vi "CameraSetting_DefaultCameraSet.vi"(7 "功能类型":enum16{"读取", "写入"}(ring), 8 "error in (no error)":errorcluster caption="错误输入（无错误）", 9 "CameraBasicInfor":string[](array[string]), 10 "字段名称":string, 11 "configuration file path":path caption="配置文件的路径") -> (0 "error out":errorcluster caption="错误输出")   [LabVIEW 2015]
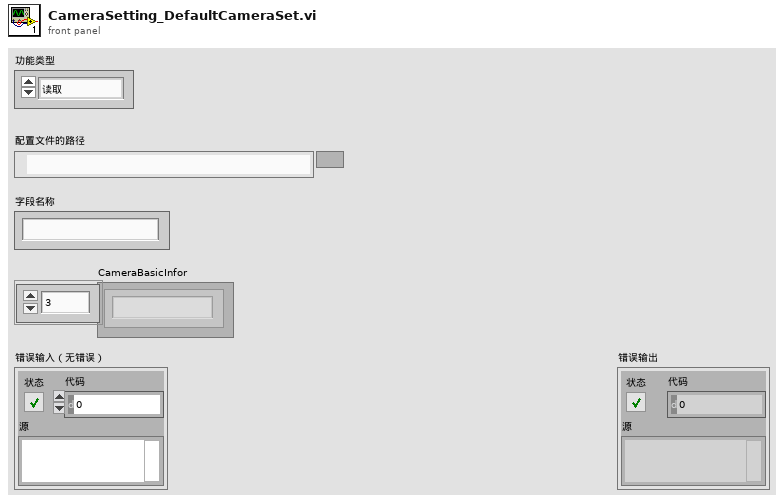
[diagram p1: front panel]
types:
  T1 = enum16{"Boolean", "DBL", "I32", "Path", "String", "U32"}
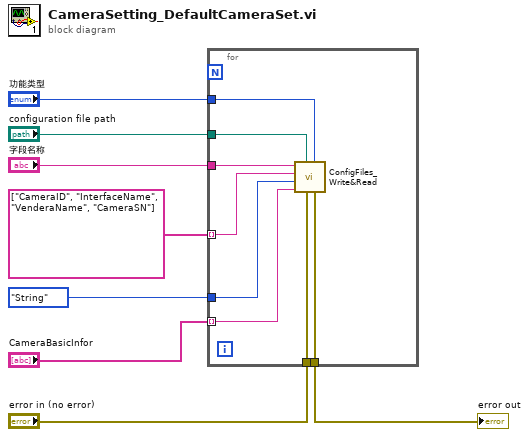
[diagram p0: block diagram]
diagram:
  n1 = for {
    tunnel: "configuration file path" -> [w16]
    tunnel: "功能类型" -> [w15]
    tunnel: "字段名称" -> [w14]
    tunnel: string[] ["CameraID", "InterfaceName", "VenderaName", "CameraSN"] -> [w13] mode=indexing
    tunnel: T1."String" ("键值类型") -> [w12]
    tunnel: "CameraBasicInfor" -> [w11] mode=indexing
    tunnel: "error in (no error)" -> [w10]
    tunnel: [w9] -> w1
    n2 = call "ConfigFiles_Write&Read.vi"("功能类型"=w15, "error in (no error)"=w10, "configuration file path"=w16, "键值_输入"=w11, "键值类型"=w12, "键名称"=w13, "字段名称"=w14) -> ("error out"=w9:errorcluster)  [unwired: 1 in, 3 out]
  }
  "error out" <- w1
